vi "Config Pulse Step Increment.vi"(0 "VISA Resource Name":refnum<visa-resource-name>, 1 "Pulse (0: UP)":i16(ring) items=["UP", "DOWN"], 2 "Pulse Step (1.0e-6)":dbl=1.0, 7 "Period (0: UP)":i16(ring) items=["UP", "DOWN"], 9 "Period Step (1.0e-6)":dbl=1.0, 11 "error in (no error)":errorcluster {"code" format="%.0x"}) -> (4 "VISA Resource Name Out":refnum<visa-resource-name>, 15 "error out":errorcluster {"code" format="%.0x"})   [LabVIEW 2012, in "Agilent ESG Series.lvlib"]
doc: "This VI configures Pulse Step Increment parameters.\n\nNotes:\n(1) This VI is supported for Agilent E4438C only."
uses:
  <instrlib>/Agilent ESG Series/Agilent ESG Series.lvlib
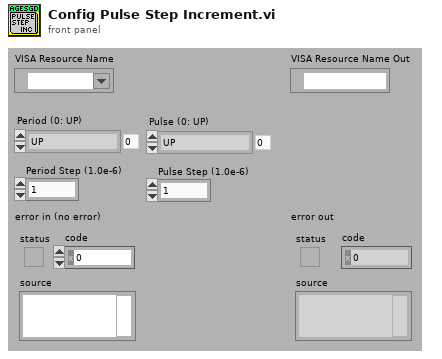
[diagram p1: front panel]
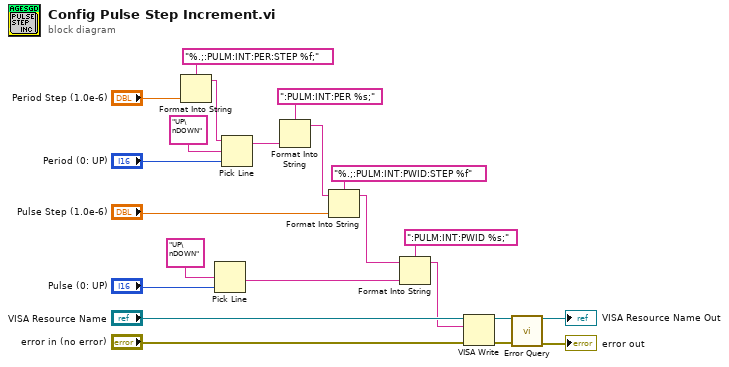
[diagram p0: block diagram]
diagram:
  n1 = Format Into String(format string="%.;:PULM:INT:PER:STEP %f;", "Period Step (1.0e-6)") -> (resulting string=w4:string)  [unwired: 2 in, 1 out]
  n2 = Pick Line(multi-line string="UP\nDOWN", line index="Pulse (0: UP)") -> (output string=w8:string)  [unwired: 1 in]
  n3 = Pick Line(string ("")=w4, multi-line string="UP\nDOWN", line index="Period (0: UP)") -> (output string=w12:string)
  n4 = Format Into String(format string=":PULM:INT:PER %s;", w12) -> (resulting string=w3:string)  [unwired: 2 in, 1 out]
  n5 = Format Into String(format string="%.;:PULM:INT:PWID:STEP %f", initial string=w3, "Pulse Step (1.0e-6)") -> (resulting string=w1:string)  [unwired: 1 in, 1 out]
  n6 = Format Into String(format string=":PULM:INT:PWID %s;", initial string=w1, w8) -> (resulting string=w2:string)  [unwired: 1 in, 1 out]
  n7 = VISA Write(VISA resource name="VISA Resource Name", write buffer=w2, error in (no error)="error in (no error)") -> (VISA resource name out=w18:refnum<visa-resource-name>, error out=w17:errorcluster)  [unwired: 1 out]
  n8 = call <instrlib>:"Error Query.vi"("VISA Resource Name"=w18, "error in (no error)"=w17) -> ("VISA Resource Name Out"=→"VISA Resource Name Out":refnum<visa-resource-name>, "error out"=→"error out":errorcluster)  [unwired: 10 in, 2 out]
